vi "Configure Link Mode.vi"(8 "error in":errorcluster, 10 "Link Mode":u16(ring) items=["OutPut", "Track", "Duplicate"], 11 "VISA resource name":refnum<visa-resource-name>) -> (0 "error out":errorcluster, 3 "VISA resource name out":refnum<visa-resource-name>)   [LabVIEW 2018, in "IT-M3100.lvlib"]
doc: "This command sets the link mode.\n<b>Link Mode</b>\n0:Output\n1:Track\n2:Duplicate"
uses:
  IT-M3100.lvlib
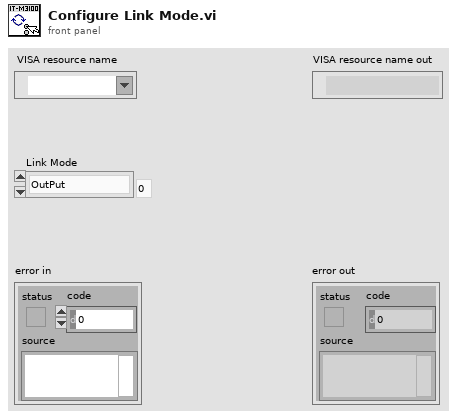
[diagram p1: front panel]
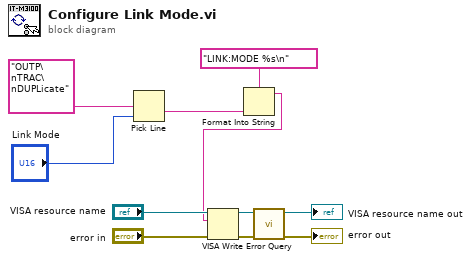
[diagram p0: block diagram]
diagram:
  n1 = Pick Line(multi-line string="OUTP\nTRAC\nDUPLicate", line index="Link Mode") -> (output string=w2:string)  [unwired: 1 in]
  n2 = Format Into String(format string="LINK:MODE %s\n", w2) -> (resulting string=w1:string)  [unwired: 2 in, 1 out]
  n3 = VISA Write(VISA resource name="VISA resource name", write buffer=w1, error in (no error)="error in") -> (VISA resource name out=w8:refnum<visa-resource-name>, error out=w9:errorcluster)  [unwired: 1 out]
  n4 = call "Error Query.vi"("error in"=w9, "VISA resource name"=w8) -> ("error out"=→"error out":errorcluster, "VISA resource name out"=→"VISA resource name out":refnum<visa-resource-name>)  [unwired: 6 in, 2 out]
